vi "RGBlezenfinaal.vi"(2 "error in (no error)":errorcluster) -> (0 "OK Button 2":bool)   [LabVIEW 2019]
uses:
  <vilib>/myRIO/Instrument Drivers/Onboard IO/I2C/typedefs/I2C Transfer Rate.ctl
  <vilib>/myRIO/Instrument Drivers/Onboard IO/I2C/I2C.lvlib
  <vilib>/myRIO/Instrument Drivers/Onboard IO/I2C/typedefs/I2C User Configuration.ctl
  <vilib>/myRIO/Instrument Drivers/Onboard IO/I2C/typedefs/I2C Configuration.ctl
  <vilib>/myRIO/Common/Instrument Driver Framework/myRIO v1.0/I2C/typedefs/I2C Channels Enum.ctl
  <vilib>/myRIO/Common/Instrument Driver Framework/Utilities/typedefs/Generic FPGA Reference.ctl
  <vilib>/myRIO/Common/Instrument Driver Framework/Utilities/typedefs/myRIO v1.0 Reference.ctl
  <vilib>/myRIO/Common/Instrument Driver Framework/Utilities/typedefs/Hardware Version Enum.ctl
  <vilib>/myRIO/Common/Instrument Driver Framework/Utilities/typedefs/myRIO Generic Hardware Reference.ctl
  <vilib>/myRIO/Instrument Drivers/Onboard IO/I2C/typedefs/I2C Reference.ctl
  <vilib>/myRIO/Instrument Drivers/Onboard IO/I2C/vis/Configure.vi
  <vilib>/myRIO/Instrument Drivers/Onboard IO/I2C/vis/Write Read.vi
  <vilib>/userDefined/High Color/nirio_resource_hc.ctl
  <vilib>/myRIO/Common/Instrument Driver Framework/myRIO v1.0/I2C/vis/myRIO v1.1 Open I2C.vi
  <vilib>/myRIO/Instrument Drivers/Onboard IO/I2C/vis/myRIO I2C Open.xnode
  <vilib>/myRIO/Common/Instrument Driver Framework/Utilities/vis/Is FPGA Ref Available.vi
  <vilib>/myRIO/Express VI/Onboard IO/I2C/I2C Express VI.xnode
  <vilib>/gmath/NI_Gmath.lvlib
panel:
  out "Eerste keer":bool
  out "Array 2":dbl[](array[numeric])
  out "High 4":u8[](array[numeric])
  out "Low 4":u8[](array[numeric])
  out "error out 3":errorcluster
  in  "Low 3":string="–"
  in  "High 3":string="—"
  out "x+y 2":u32
  out "x+y":u32
  out "Array":dbl[](array[numeric])
  out "spread value":dbl
  in  "stop":bool
  in  "High":string="—"
  in  "Low":string="–"
  out "error out 2":errorcluster
  out "Low 2":u8[](array[numeric])
  out "High 2":u8[](array[numeric])
  # "RED: 96, 97"
  # "GREEN: 98, 99"
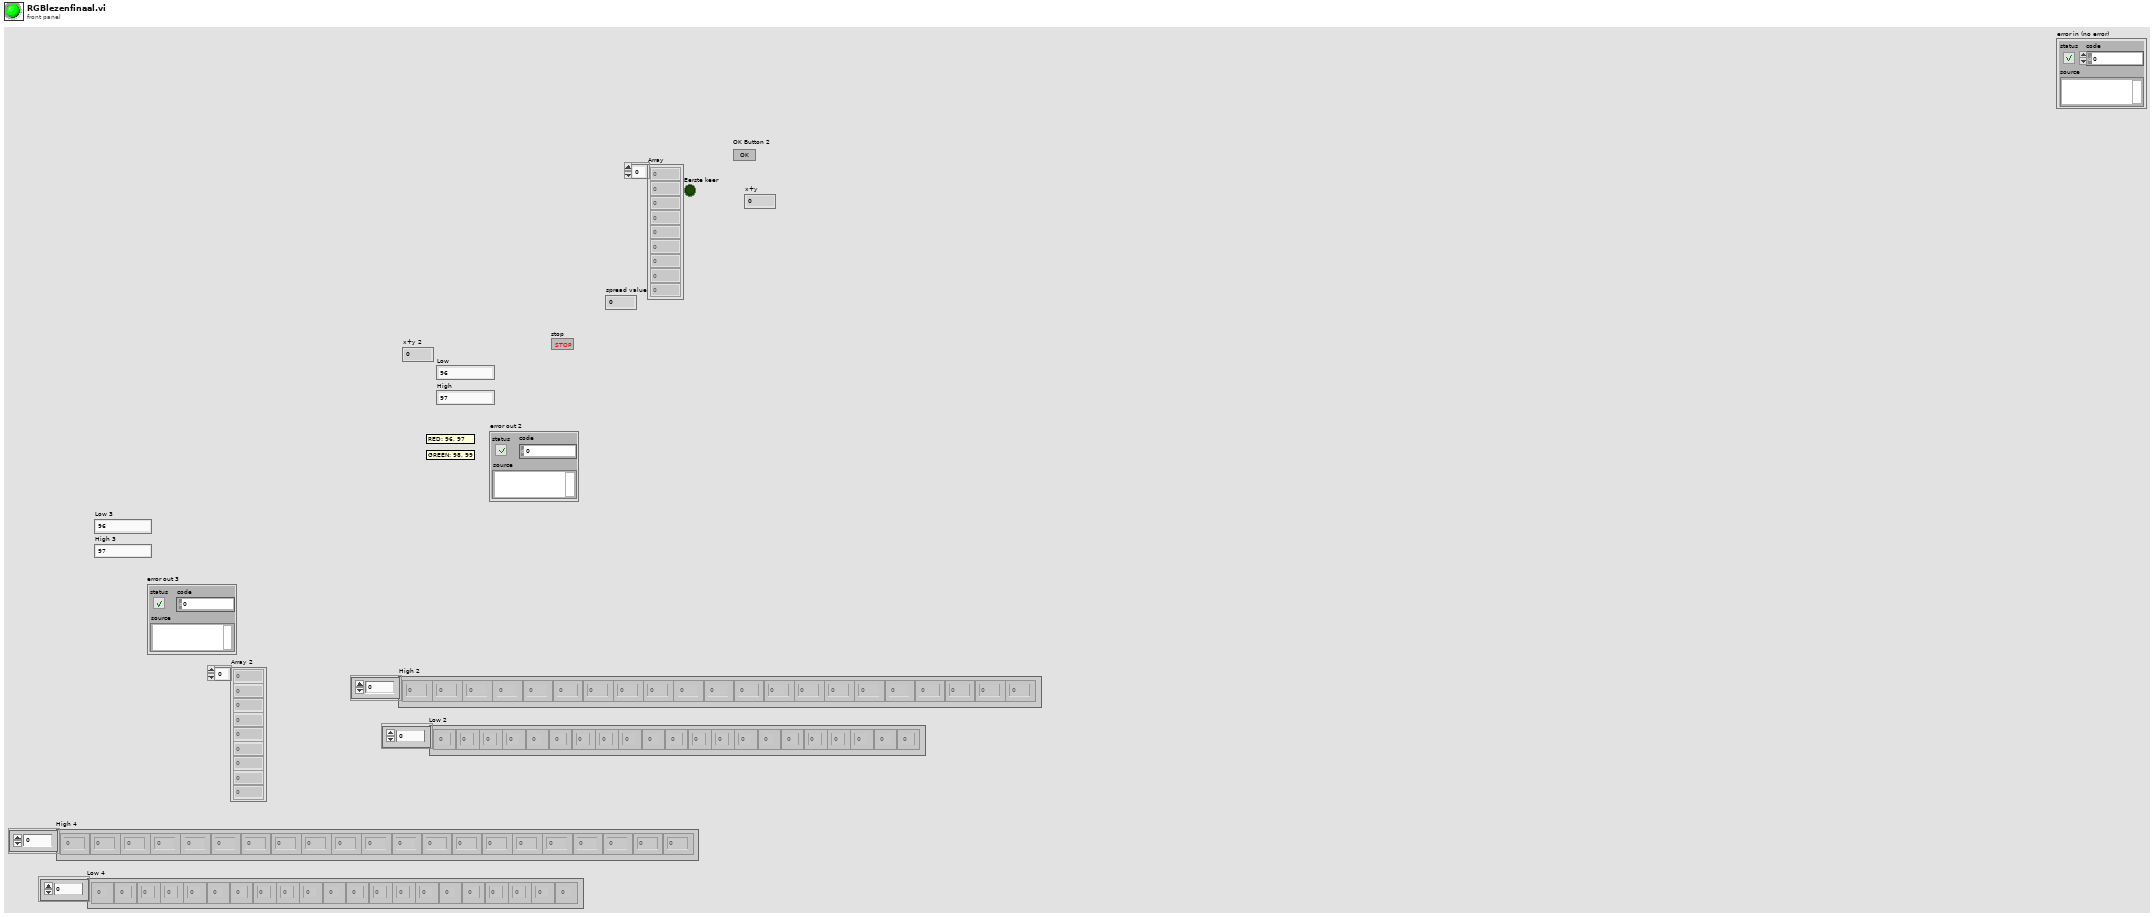
[diagram p1: front panel]
types:
  T1 = typedef "I2C.lvlib/I2C Reference.ctl" = cluster{"myRIO Reference":T2, "I2C Channels Enum":T6, "I2C Configuration":T7}
  T2 = typedef "myRIO Generic Hardware Reference.ctl" = cluster{"myRIO Model":T3, "myRIO Hardware Reference":T4}
  T3 = typedef "Hardware Version Enum.ctl" = enum16{"Unknown", "myRIO-1900", "myRIO-1950", "roboRIO", "NI ELVIS RIO CM", "ELVIS III"}
  T4 = typedef "myRIO v1.0 Reference.ctl" = cluster{"Generic FPGA Reference":T5, "Allow multiple opens":bool}
  T5 = typedef "Generic FPGA Reference.ctl" = refnum<k20>
  T6 = typedef "I2C Channels Enum.ctl" = enum16{"Not Connected", "A/I2C", "B/I2C", "I2C/I2C"}
  T7 = typedef "I2C.lvlib/I2C Configuration.ctl" = cluster{"I2C Transfer Rate":T8}
  T8 = typedef "I2C.lvlib/I2C Transfer Rate.ctl" = enum16{"Standard mode (100 kbps)", "Fast mode (400 kbps)"}
  T9 = typedef "I2C.lvlib/I2C User Configuration.ctl" = cluster{"I2C Transfer Rate":T8}
  T10 = typedef "nirio_resource_hc.ctl" = tag
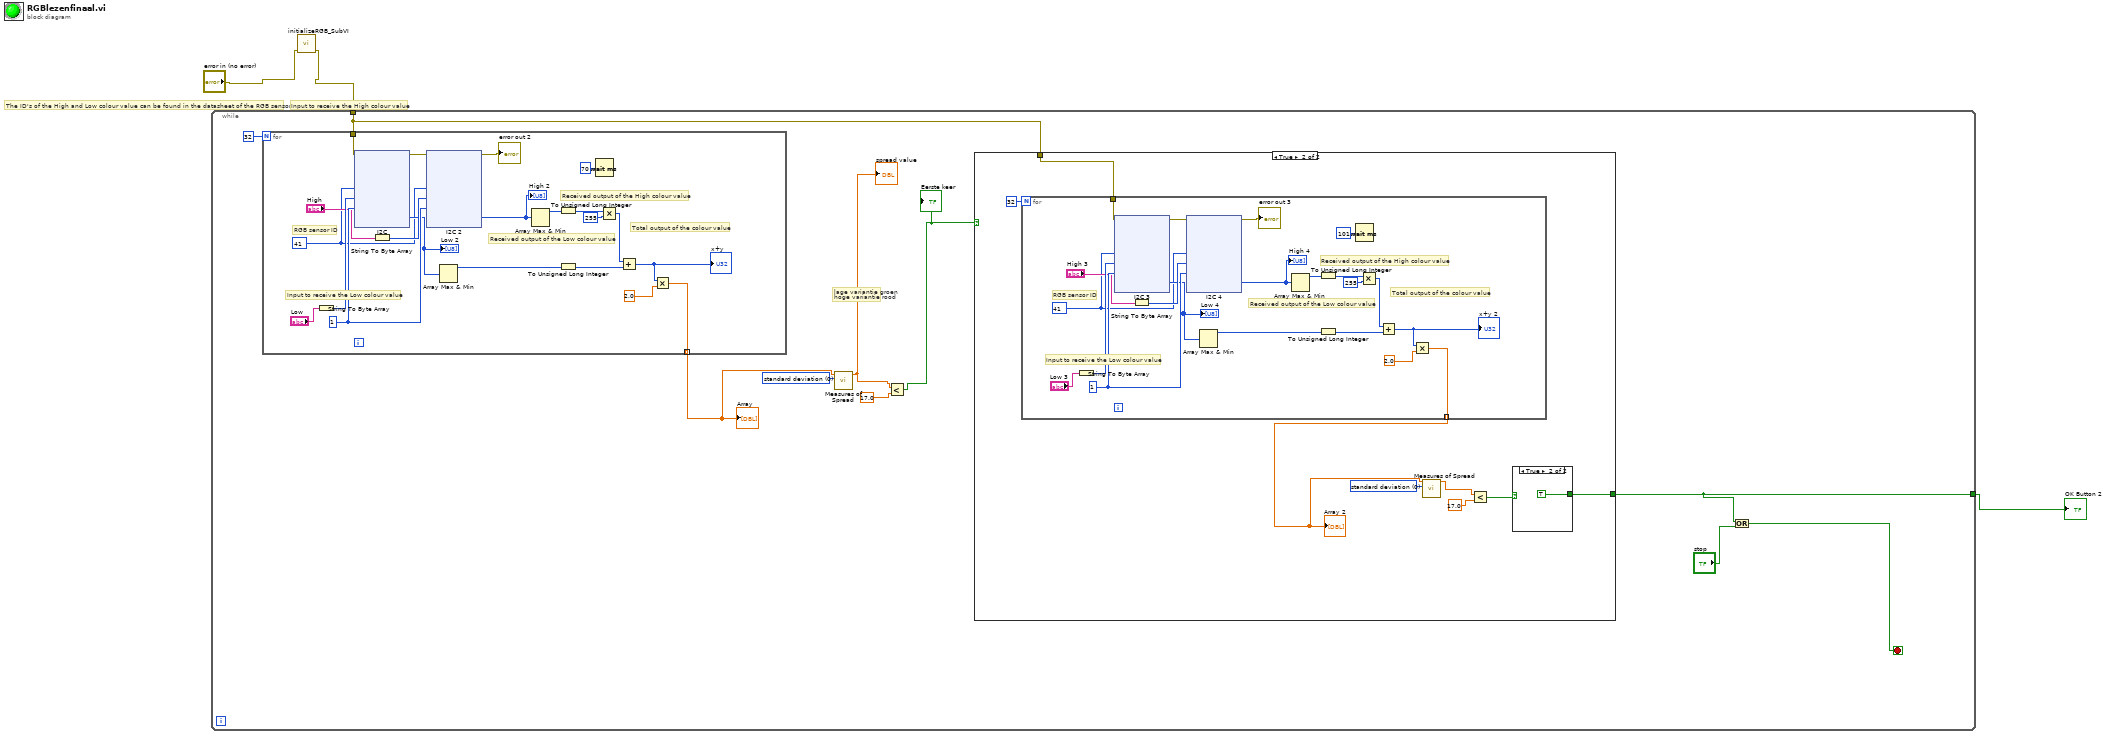
[diagram p0: block diagram]
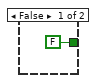
[diagram p2: hidden frame]
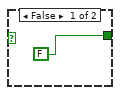
[diagram p3: hidden frame]
diagram:
  # "The ID's of the High and Low colour value can be found in the datasheet of the RGB sensor"
  # "Input to receive the High colour value"
  n1 = call "initializeRGB_SubVI.vi"("error in (no error)"="error in (no error)") -> ("error out"=w2:errorcluster)  [unwired: 10 in]
  n2 = while {
    tunnel: w2 -> [w10]
    tunnel: [w9] -> w1
    stop <- w7 stop-if-true
    w13 = 0 items=["standard deviation", "range", "mean absolute deviation", "interquartile range"] ("type")
    # "lage variantie groen\nhoge variantie rood"
    n3 = for {
      N: 32 -> [_]
      tunnel: w10 -> [w18]
      tunnel: [w14] -> w11 mode=indexing
      w19 = 41 ("Numeric")
      w31 = u32 1 ("Byte Count")
      # "Total output of the colour value"
      # "Received output of the Low colour value"
      # "Received output of the High colour value"
      # "Input to receive the Low colour value"
      # "RGB sensor ID"
      n4 = String To Byte Array(string="Low") -> (unsigned byte array=w30:u8[])
      n5 = xnode "I2C"("Slave Address (7-bit)"=w19, "Bytes to Write"=w30, "Byte Count"=w31, "error in (no error)"=w18) -> ("Bytes Read"=w27:u8[], "error out"=w32:errorcluster)
      "Low 2" <- w27
      n6 = String To Byte Array(string="High") -> (unsigned byte array=w29:u8[])
      n7 = xnode "I2C 2"("Slave Address (7-bit)"=w19, "Bytes to Write"=w29, "Byte Count"=w31, "error in (no error)"=w32) -> ("Bytes Read"=w26:u8[], "error out"=→"error out 2":errorcluster)
      "High 2" <- w26
      n8 = Array Max & Min(array=w27) -> (max value=w21:u8)  [unwired: 3 out]
      n9 = Array Max & Min(array=w26) -> (max value=w23:u8)  [unwired: 3 out]
      n10 = To Unsigned Long Integer(number=w23) -> (unsigned 32bit integer=w22:u32)
      n11 = To Unsigned Long Integer(number=w21) -> (unsigned 32bit integer=w20:u32)
      n12 = Wait (ms)(milliseconds to wait=u32 70) -> ()  [unwired: 1 out]
      n13 = Multiply(x=w22, y=u32 255) -> (x*y=w24:u32)
      n14 = Add(x=w24, y=w20) -> (x+y=w16:u32)
      "x+y" <- w16
      n15 = Multiply(x=w16, y=2.0) -> (x*y=w14:dbl)
    }
    "Array" <- w11
    n16 = call <vilib>:"Measures of Spread.vi"("type"=w13, "x array"=w11) -> ("spread value"=w6:dbl)  [unwired: 8 in, 1 out]
    "spread value" <- w6
    n17 = Less?(x=w6, y=17.0) -> (x < y?=w5:bool)
    "Eerste keer" <- w5
    n18 = case shown="True" w5 {
      tunnel: w10 -> [_ w123]
      tunnel: [FALSE w120] -> w9
      frame False {
      }
      frame True {
        w122 = 0 items=["standard deviation", "range", "mean absolute deviation", "interquartile range"] ("type")
        n19 = for {
          N: 32 -> [_]
          tunnel: w123 -> [w130]
          tunnel: [w126] -> w121 mode=indexing
          w131 = 41 ("Numeric")
          w143 = u32 1 ("Byte Count")
          # "Total output of the colour value"
          # "Received output of the Low colour value"
          # "Received output of the High colour value"
          # "Input to receive the Low colour value"
          # "RGB sensor ID"
          n20 = String To Byte Array(string="Low 3") -> (unsigned byte array=w142:u8[])
          n21 = xnode "I2C 3"("Slave Address (7-bit)"=w131, "Bytes to Write"=w142, "Byte Count"=w143, "error in (no error)"=w130) -> ("Bytes Read"=w139:u8[], "error out"=w144:errorcluster)
          "Low 4" <- w139
          n22 = String To Byte Array(string="High 3") -> (unsigned byte array=w141:u8[])
          n23 = xnode "I2C 4"("Slave Address (7-bit)"=w131, "Bytes to Write"=w141, "Byte Count"=w143, "error in (no error)"=w144) -> ("Bytes Read"=w138:u8[], "error out"=→"error out 3":errorcluster)
          "High 4" <- w138
          n24 = Array Max & Min(array=w139) -> (max value=w133:u8)  [unwired: 3 out]
          n25 = Array Max & Min(array=w138) -> (max value=w135:u8)  [unwired: 3 out]
          n26 = To Unsigned Long Integer(number=w135) -> (unsigned 32bit integer=w134:u32)
          n27 = To Unsigned Long Integer(number=w133) -> (unsigned 32bit integer=w132:u32)
          n28 = Wait (ms)(milliseconds to wait=u32 101) -> ()  [unwired: 1 out]
          n29 = Multiply(x=w134, y=u32 255) -> (x*y=w136:u32)
          n30 = Add(x=w136, y=w132) -> (x+y=w128:u32)
          "x+y 2" <- w128
          n31 = Multiply(x=w128, y=2.0) -> (x*y=w126:dbl)
        }
        "Array 2" <- w121
        n32 = call <vilib>:"Measures of Spread.vi"("type"=w122, "x array"=w121) -> ("spread value"=w117:dbl)  [unwired: 8 in, 1 out]
        n33 = Less?(x=w117, y=17.0) -> (x < y?=w116:bool)
        n34 = case shown="True" w116 {
          tunnel: [FALSE TRUE] -> w120
          frame False {
          }
          frame True {
          }
        }
      }
    }
    n35 = Or(x=w9, y="stop") -> (x .or. y?=w7:bool)
  }
  "OK Button 2" <- w1
